vi "Stop Loops--Global Variable.vi"() -> ()   [LabVIEW 2020, in "global_stop_flag.lvlib"]
doc: "The purpose of this global variable is to provide a means for the application to quickly stop all loops.\n\nFor example, imagine a state machine takes 10 seconds to loop and executes all its states. The user starts the state machine. After 1 second, the user presses the \"Abort\" button.\n\nThe loop of this state machine can poll this global variable. Thus, the loop can stop soon after the user presses \"Abort\". PT, 23 October 2019"
uses:
  global_stop_flag.lvlib
panel:
  in  "Stop all loops?":bool
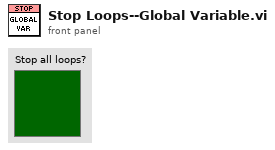
[diagram p1: front panel]
diagram:
